vi "ASI_bufferToImage.vi"(0 "iWidth":i32, 5 "iHeight":i32, 7 "New Image":T1, 9 "imageType":i32, 11 "pBuffer in":u8[](array[numeric])) -> (4 "Image":T1(plugin-control))   [LabVIEW 2023]
uses:
  <vilib>/vision/Image Controls.llb/IMAQ Image.ctl
panel:
  in  "16bit type 2":u16[](array[numeric])
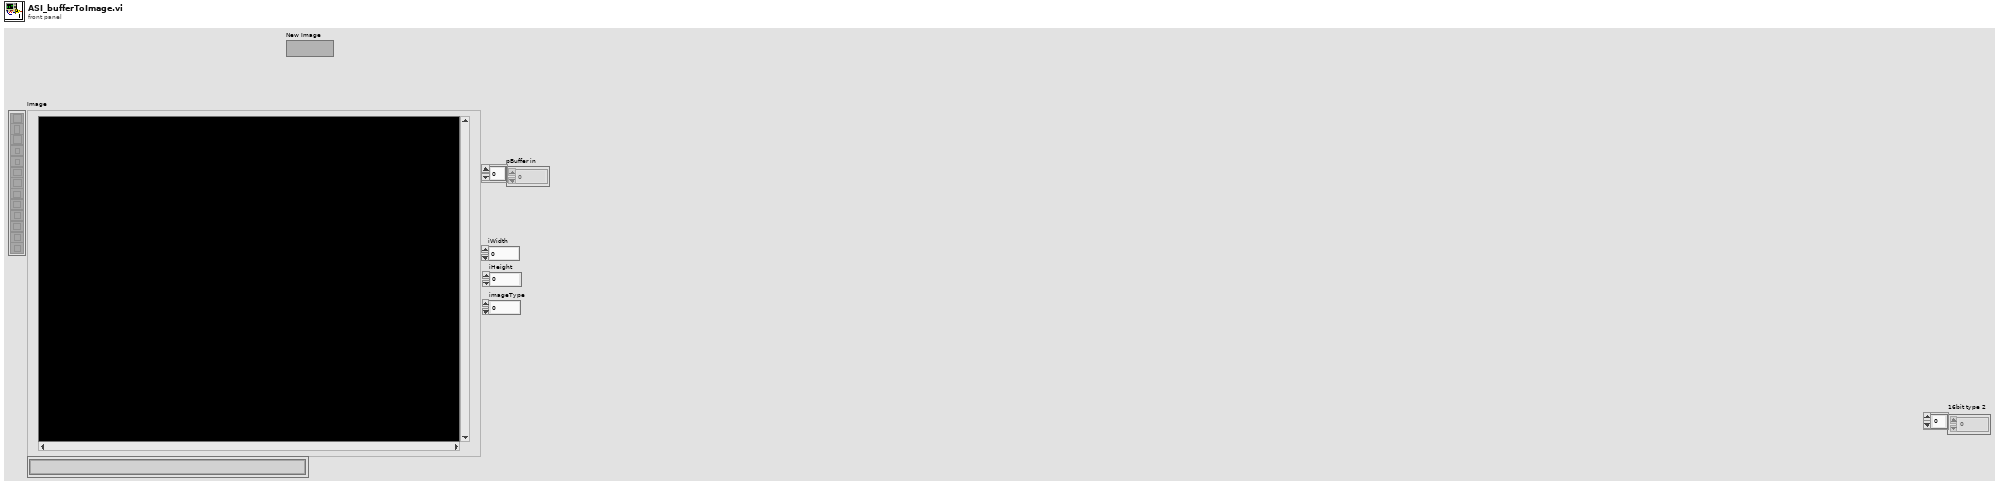
[diagram p1: front panel]
types:
  T1 = typedef "IMAQ Image.ctl" = refnum<image>
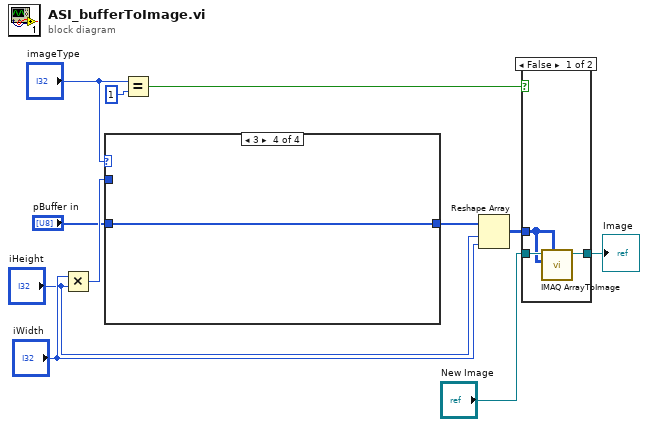
[diagram p0: block diagram]
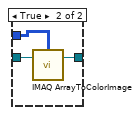
[diagram p2: hidden frame]
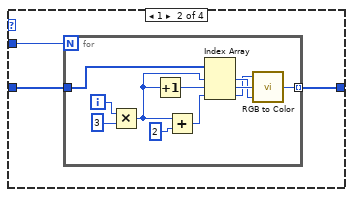
[diagram p4: hidden frame]
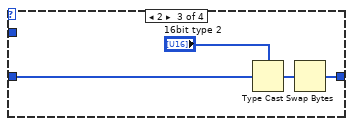
[diagram p5: hidden frame]
diagram:
  n1 = Multiply(x="iWidth", y="iHeight") -> (x*y=w11:i32)
  n2 = case shown="3" "imageType" {
    tunnel: [w12 w13 w27 w31] -> w6
    tunnel: "pBuffer in" -> [w12 w14 w28 w31]
    tunnel: w11 -> [_ w15 _ _]
    frame 0, Default {
    }
    frame 1 {
      n3 = for {
        N: w15 -> [_]
        tunnel: w14 -> [w25]
        tunnel: [w20] -> w13 mode=indexing
        i -> [w18]
        n4 = Multiply(x=w18, y=u16 3) -> (x*y=w19:i32)
        n5 = Increment(x=w19) -> (x+1=w24:i32)
        n6 = Add(x=w19, y=2 ("x")) -> (x+y=w23:i32)
        n7 = Index Array(array=w25, index #1=w19, index #2=w24, index #3=w23) -> (element #1=w17:u8, element #2=w21:u8, element #3=w16:u8)
        n8 = call <vilib>:"RGB to Color.vi"("B"=w17, "G"=w21, "R"=w16) -> ("Color"=w20:u32)
      }
    }
    frame 2 {
      n9 = Type Cast(type="16bit type 2", x=w28) -> (*(type *) &x=w29:u16[])
      n10 = Swap Bytes(anything=w29) -> (byte swapped=w27:u16[])
    }
    frame 3 {
    }
  }
  n11 = Equal?(x="imageType", y=u8 1) -> (x = y?=w9:bool)
  n12 = Reshape Array(w6, "iHeight", "iWidth") -> (w7:u32[][])
  n13 = case shown="False" w9 {
    tunnel: w7 -> [w32 w37]
    tunnel: "New Image" -> [w34 w35]
    tunnel: [w33 w36] -> w8
    frame False {
      n14 = call "IMAQ ArrayToImage"("Image Pixels (U16)"=w32, "Image Pixels (U8)"=w32, "Image"=w34) -> ("Image Out"=w33:T1)  [unwired: 7 in, 1 out]
    }
    frame True {
      n15 = call "IMAQ ArrayToColorImage"("Image Pixels (U32)"=w37, "Image"=w35) -> ("Image Out"=w36:T1)  [unwired: 3 in, 1 out]
    }
  }
  "Image" <- w8
